vi "UI_AR_Do_Rank0Special.vi"(8 "error in (no error)":errorcluster, 9 "Parameters":T1={"Write TipStrips with details (T)"=TRUE, "Write Captions with UserLabels (T)"=TRUE, "Mode (ind only)"=enum."Indicators only", "Enable nested stream (T)"=TRUE}, 10 "Databox_sealed":refnum<class "Databox_sealed.lvclass">, 11 "UI_Actor in":refnum<class "UI_Actor.lvclass">) -> (0 "error out":errorcluster, 3 "UI_Actor out":refnum<class "UI_Actor.lvclass">)   [LabVIEW 2020, in "UI_Actor.lvlib" / "UI_Actor.lvclass"]
uses:
  UI_Actor.lvclass
  ctl_AR_Parameters.ctl
  ctl_AR_Mode.ctl
  support/Databox.lvlibp/Databox_sealed/Databox_sealed.lvclass
  D:/Projets/STEP AT/UI Actor/support/Databox.lvlibp/Databox/Databox.lvclass
  UI_Actor.lvclass/UI_Actor.ctl
  <vilib>/Utility/miscctls.llb/LVMapReplaceAction.ctl
  support/Databox.lvlibp/Databox/Read Builder name.vi
  support/Databox.lvlibp/Databox/Databox.lvclass
  D:/Projets/STEP AT/UI Actor/support/Databox.lvlibp/Databox_sealed/Databox_sealed.lvclass
  support/Databox.lvlibp/TypesTools/Config/Config.lvclass
  support/Databox.lvlibp/TypesTools/Data/Data.lvclass
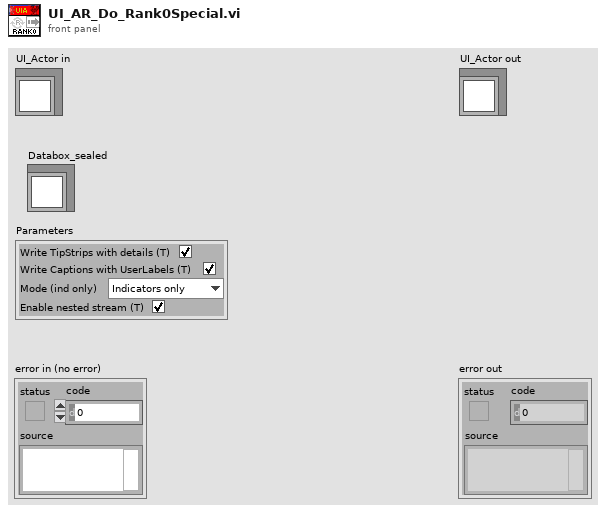
[diagram p1: front panel]
types:
  T1 = typedef "UI_Actor.lvlib/UI_Actor.lvclass/ctl_AR_Parameters.ctl" = cluster{"Write TipStrips with details (T)":bool, "Write Captions with UserLabels (T)":bool, "Mode (ind only)":T2, "Enable nested stream (T)":bool}
  T2 = typedef "UI_Actor.lvlib/UI_Actor.lvclass/ctl_AR_Mode.ctl" = enum16{"Controls only", "Indicators only", "All"}
  T3 = typedef "LVMapReplaceAction.ctl" = enum32{"Modify Entry only if found", "Add or Modify Entry", "Delete Entry"}
  T4 = typedef "UI_Actor.lvlib/UI_Actor.lvclass/ctl_InternalMapItem.ctl" = cluster{"Config":refnum<class "Config.lvclass">, "LatestData":refnum<class "Data.lvclass">}
  T5 = cluster{"Conf":refnum<class "Config.lvclass">, "Latest Data":refnum<class "Data.lvclass">}
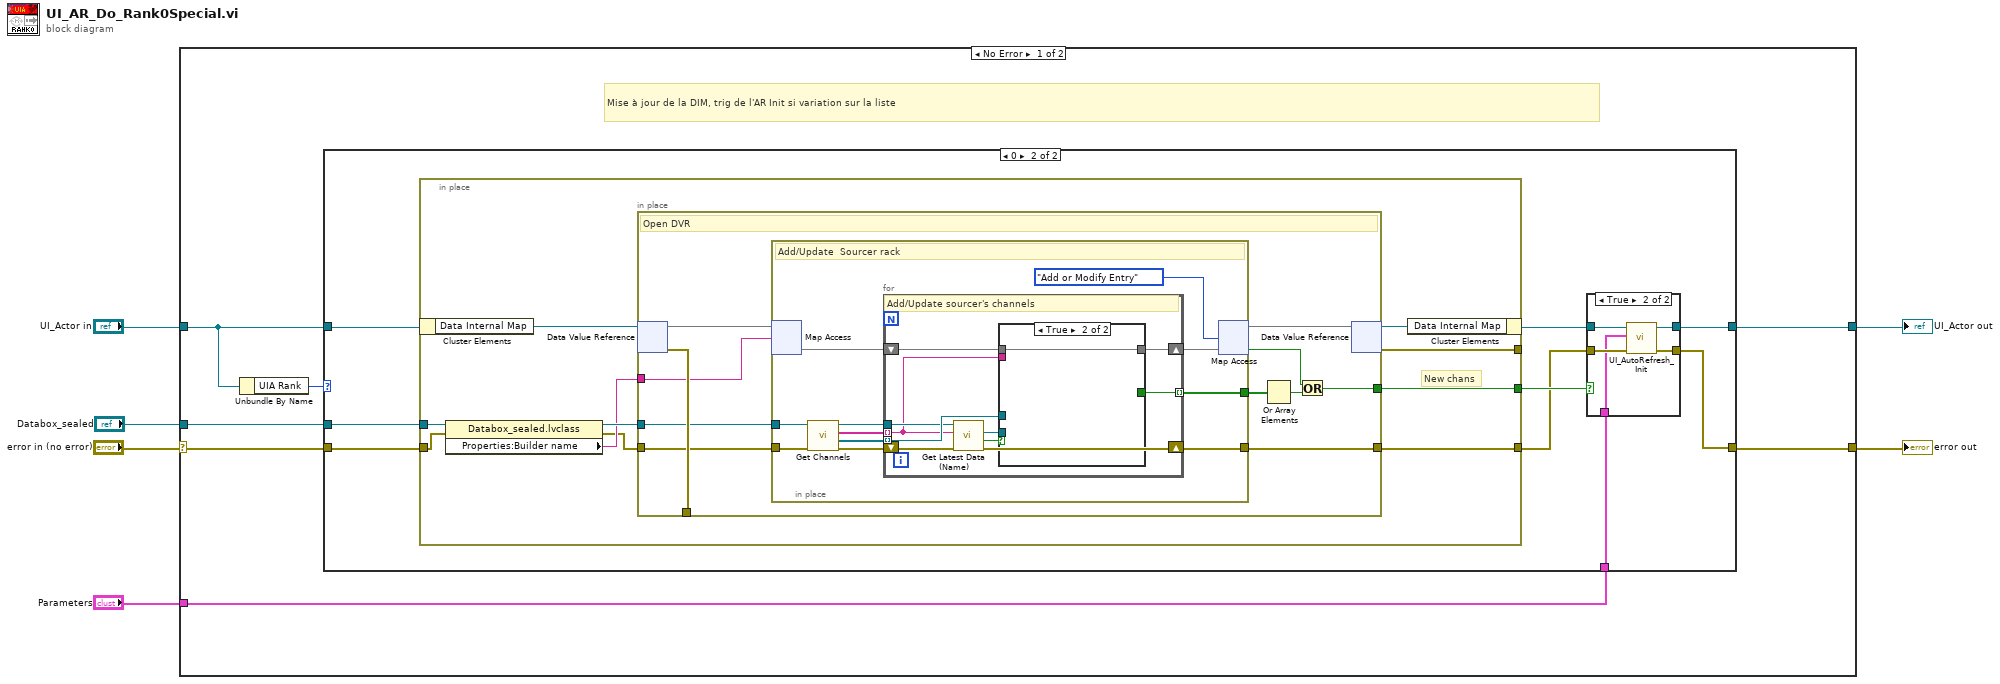
[diagram p0: block diagram]
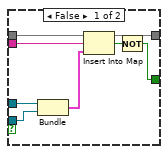
[diagram p3: hidden frame]
diagram:
  n1 = case shown="No Error" "error in (no error)" {
    selector: "error in (no error)" -> [w9 w84]
    tunnel: [w10 w84] -> w5
    tunnel: [w11 w83] -> w3
    tunnel: "UI_Actor in" -> [w12 w83]
    tunnel: "Parameters" -> [w7 _]
    tunnel: "Databox_sealed" -> [w8 _]
    frame No Error {
      # "Mise à jour de la DIM, trig de l'AR Init si variation sur la liste"
      n2 = Unbundle By Name(w12) -> ("UIA Rank"=w13:i32)
      n3 = case shown="0" w13 {
        tunnel: [w15 w22] -> w11
        tunnel: w12 -> [w15 w24]
        tunnel: [w14 w20] -> w10
        tunnel: w9 -> [w14 w17]
        tunnel: w8 -> [_ w16]
        tunnel: w7 -> [_ w18]
        frame Default {
        }
        frame 0 {
          n4 = in-place {
            in-place-border: [w32] -> _
            in-place-border: [w30] -> w21
            in-place-border: [w31] -> w19
            in-place-border: w17 -> [w25]
            in-place-border: w16 -> [w29]
            # "New chans"
            n5 = in-place-cluster #1(w24) -> ("Data Internal Map"=w34:refnum<data-value>)
            n6 = property class="Databox_sealed.lvclass"(reference=w29, error in=w25) -> (reference out=w28:refnum<class "Databox_sealed.lvclass">, error out=w26:errorcluster, "Properties:Builder name"=w27:string)
            n7 = in-place {
              in-place-border: [w45] -> _
              in-place-border: [w43] -> w31
              in-place-border: [w36] -> w30
              in-place-border: w26 -> [w42]
              in-place-border: w28 -> [w41]
              in-place-border: w27 -> [w35]
              # "Open DVR"
              n8 = in-place-dvr #2(w34) -> (w40:map{string, map{string, T4}}, w45:errorcluster)
              n9 = in-place {
                in-place-border: [w56] -> w44
                in-place-border: [w55] -> w43
                in-place-border: w42 -> [w54]
                in-place-border: w41 -> [w53]
                # "Add/Update  Sourcer rack"
                n10 = in-place-map #3(w40, w35) -> (w48:map{string, T4})  [unwired: 1 in, 1 out]
                n11 = call "Get Channels.vi"("error in (no error)"=w54, "Databox in"=w53) -> ("error out"=w52:errorcluster, "Channels configs."=w51:refnum<class "Config.lvclass">[], "Channels names"=w50:string[], "Databox out"=w49:refnum<class "Databox_sealed.lvclass">)  [unwired: 6 in]
                n12 = for {
                  tunnel: w50 -> [w59] mode=indexing
                  tunnel: w51 -> [w65] mode=indexing
                  tunnel: w49 -> [w63]
                  tunnel: [w57] -> w56 mode=indexing
                  shift-right: [w61] -> w47
                  shift-left: w48 -> [w66]
                  shift-right: [w60] -> w55
                  shift-left: w52 -> [w62]
                  # "Add/Update sourcer's channels"
                  n13 = call "Get Latest Data (Name).vi"("error in (no error)"=w62, "Node Name"=w59, "Databox in"=w63) -> ("error out"=w60:errorcluster, "Data empty!"=w58:bool, "Latest Data"=w64:refnum<class "Data.lvclass">)  [unwired: 5 in, 1 out]
                  n14 = case shown="True" w58 {
                    tunnel: w66 -> [w74 w75]
                    tunnel: w65 -> [w73 _]
                    tunnel: w64 -> [w72 _]
                    tunnel: [w71 w75] -> w61
                    tunnel: w59 -> [w70 _]
                    tunnel: [w67 _] -> w57
                    frame False {
                      n15 = Bundle("Conf"=w73, "Latest Data"=w72) -> (w69:T5)  [unwired: 1 in]
                      n16 = Insert Into Map(map in=w74, key=w70, value=w69) -> (map out=w71:map{string, T4}, key already included?=w68:bool)  [unwired: 1 out]
                      n17 = Not(x=w68) -> (.not. x?=w67:bool)
                    }
                    frame True {
                    }
                  }
                }
                n18 = in-place-map #3(w47, LVMapReplaceAction."Add or Modify Entry" ("action")) -> (w39:map{string, map{string, T4}}, w38:bool)  [unwired: 1 out]
              }
              n19 = Or Array Elements(Boolean array=w44) -> (logical OR=w37:bool)
              n20 = Or(x=w38, y=w37) -> (x .or. y?=w36:bool)
              n21 = in-place-dvr #2(w39) -> (w33:refnum<data-value>, w32:errorcluster)
            }
            n22 = in-place-cluster #1("Data Internal Map"=w33) -> (w23:refnum<class "UI_Actor.lvclass">)
          }
          n23 = case shown="True" w21 {
            tunnel: w23 -> [w77 w82]
            tunnel: [w77 w81] -> w22
            tunnel: [w76 w80] -> w20
            tunnel: w19 -> [w76 w79]
            tunnel: w18 -> [_ w78]
            frame False {
            }
            frame True {
              n24 = call-dynamic "UI_AutoRefresh_Init.vi"("error in (no error)"=w79, "Parameters"=w78, "UI_Actor in"=w82) -> ("error out"=w80:errorcluster, "UI_Actor out"=w81:refnum<class "UI_Actor.lvclass">)  [unwired: 7 in]
            }
          }
        }
      }
    }
    frame Error {
    }
  }
  "error out" <- w5
  "UI_Actor out" <- w3
